vi "扭矩1.vi"() -> ()   [LabVIEW 2020]
uses:
  <userlib>/DAQNavi Polymorphic VI/create/DAQNavi Create Channel(AI-Voltage).vi
  Global_Variable/Global.vi
  <userlib>/DAQNavi Polymorphic VI/read/DAQNavi Read (Analog 1D DBL NChan 1Samp).vi
panel:
  out "簇":cluster{"左加载":dbl, "右加载":dbl}
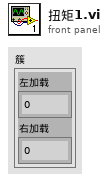
[diagram p1: front panel]
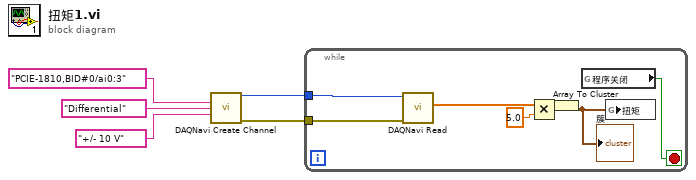
[diagram p0: block diagram]
diagram:
  n1 = call-poly <userlib>:"DAQNavi Create Channel.vi"("physical channels"="PCIE-1810,BID#0/ai0:3", "signal type"="Differential", "value range"="+/- 10 V") -> ("task out"=w3:i32, "error out"=w2:errorcluster)  [unwired: 11 in]
  n2 = while {
    tunnel: w3 -> [w12]
    tunnel: w2 -> [w11]
    stop <- w8 stop-if-true
    n3 = call-poly <userlib>:"DAQNavi Read.vi"("error in (no error)"=w11, "task in"=w12) -> ("data"=w10:dbl[])  [unwired: 7 in, 2 out]
    n4 = Multiply(x=w10, y=5.0) -> (x*y=w7:dbl[])
    n5 = Array To Cluster(array=w7) -> (cluster=w6:cluster{"[0]":dbl, "[1]":dbl})
    "簇" <- w6
    n6 = global read "Global.vi" "程序关闭"() -> (w8:bool)
    n7 = global write "Global.vi" "扭矩"(w6) -> ()
  }
